vi "ResetDAC_1212.vi"(2 "error in (no error)":errorcluster, 3 "FPGA Interface In":refnum<k20>, 4 "Selected DAC":u8(ring) items=["DAC0 (A)", "DAC1 (B)"]) -> (0 "error out":errorcluster, 1 "FPGA Interface Out":refnum<k20>)   [LabVIEW 2018]
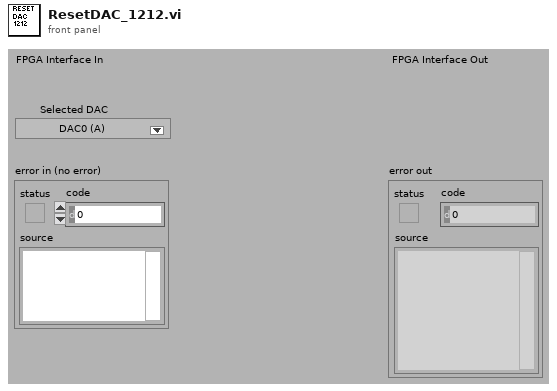
[diagram p1: front panel]
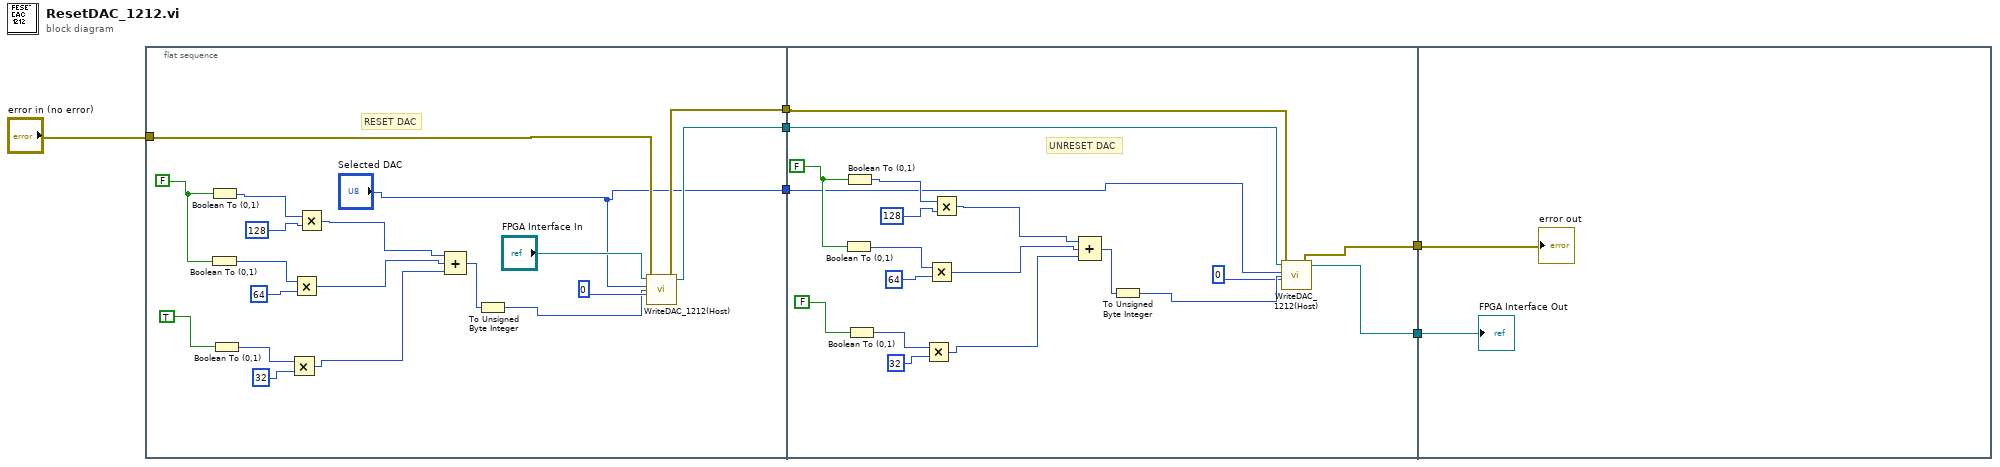
[diagram p0: block diagram]
diagram:
  n1 = flat-sequence {
    tunnel: [w25] -> w6
    tunnel: [w24] -> w5
    tunnel: "error in (no error)" -> [w9]
    tunnel: ["Selected DAC"] -> w1
    tunnel: w6 -> [w28]
    tunnel: w5 -> [w27]
    tunnel: [w30] -> w4
    tunnel: [w29] -> w3
    tunnel: w1 -> [w26]
    tunnel: w4 -> [w46]
    tunnel: w3 -> [w45]
    frame #0 {
      w11 = FALSE ("Boolean")
      # "RESET DAC"
      n2 = Boolean To (0,1)(Boolean=w11) -> (0, 1=w17:i16)
      n3 = Boolean To (0,1)(Boolean=w11) -> (0, 1=w18:i16)
      n4 = Boolean To (0,1)(Boolean=TRUE) -> (0, 1=w14:i16)
      n5 = Multiply(x=w14, y=u8 32 ("RegAddress")) -> (x*y=w12:i16)
      n6 = Multiply(x=w17, y=u8 64 ("RegAddress")) -> (x*y=w13:i16)
      n7 = Multiply(x=w18, y=u8 128 ("RegAddress")) -> (x*y=w19:i16)
      n8 = Compound Arithmetic op=unknown(w19, w13, w12) -> (w20:i16)
      n9 = To Unsigned Byte Integer(number=w20) -> (unsigned 8bit integer=w21:u8)
      n10 = call "WriteDAC_1212(Host).vi"("FPGA Interface In"="FPGA Interface In", "Selected DAC"="Selected DAC", "Address"=u8 0 ("RegAddress"), "error in (no error)"=w9, "Data"=w21) -> ("FPGA Interface Out"=w24:refnum<k20>, "error out"=w25:errorcluster)  [unwired: 1 in]
    }
    frame #1 {
      w43 = FALSE ("Boolean")
      # "UNRESET DAC"
      n11 = Boolean To (0,1)(Boolean=w43) -> (0, 1=w37:i16)
      n12 = Boolean To (0,1)(Boolean=w43) -> (0, 1=w36:i16)
      n13 = Boolean To (0,1)(Boolean=FALSE) -> (0, 1=w40:i16)
      n14 = Multiply(x=w40, y=u8 32 ("RegAddress")) -> (x*y=w42:i16)
      n15 = Multiply(x=w37, y=u8 64 ("RegAddress")) -> (x*y=w41:i16)
      n16 = Multiply(x=w36, y=u8 128 ("RegAddress")) -> (x*y=w35:i16)
      n17 = Compound Arithmetic op=unknown(w35, w41, w42) -> (w34:i16)
      n18 = To Unsigned Byte Integer(number=w34) -> (unsigned 8bit integer=w33:u8)
      n19 = call "WriteDAC_1212(Host).vi"("FPGA Interface In"=w27, "Selected DAC"=w26, "Address"=u8 0 ("RegAddress"), "error in (no error)"=w28, "Data"=w33) -> ("FPGA Interface Out"=w29:refnum<k20>, "error out"=w30:errorcluster)  [unwired: 1 in]
    }
    frame #2 {
      "error out" <- w46
      "FPGA Interface Out" <- w45
    }
  }
